vi "Sort Fcurve fxp.vi"(0 "reference in":refnum<class "Fcurve.lvclass">, 2 "Interleaved data in":fxp<+/-,27,5>[](array[numeric]), 5 "error in (no error)":errorcluster) -> (7 "Fcurve out":cluster{"X":dbl[], "Y":dbl[]}[](graph), 14 "reference out":refnum<class "Fcurve.lvclass">, 16 "Interleaved data out":fxp<+/-,27,5>[](array[numeric]), 19 "error out":errorcluster)   [LabVIEW 2019, in "Fcurve.lvclass"]
doc: "Sorts interleaved data into Fcurve"
uses:
  Fcurve.lvclass
  TDMS_DataHandler_class/property name combo box.ctl
  TDMS_DataHandler_class/TDMS_DataHandler.lvclass
panel:
  out "Ret_in":i32
  out "Con_in":i32
  out "App_in":i32
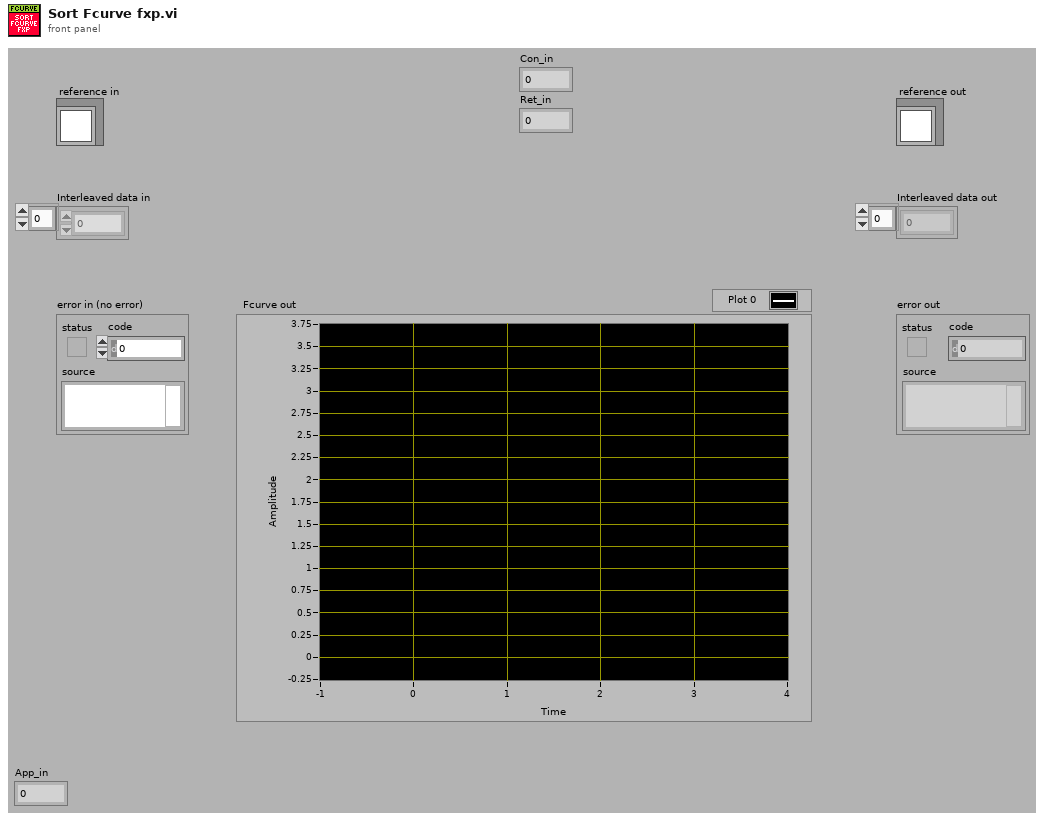
[diagram p1: front panel]
types:
  T1 = typedef "TDMS_DataHandler.lvclass/property name combo box.ctl" = string
  T2 = typedef "Fcurve.lvclass/ObjectAttributes.ctl" = cluster{"MyAttribute":dbl, "Fcurve Metadata":T3, "Contact Spread of dev":dbl, "Tau Delay (ms)":dbl, "Points of contact":dbl, "Def_wfm":cluster{"Max":dbl, "Min":dbl}, "Zpos_wfm":cluster{"Max":dbl, "Min":dbl}, "Contact stat?":bool, "Real AI dt (s)":dbl, "Decimation":cluster{"App":cluster{"Dec":i32, "apply":bool}, "Con":cluster{"Dec":i32, "apply":bool}, "Ret":cluster{"Dec":i32, "apply":bool}}, "Segment def[0]":dbl, "Segment Zpos[0]":dbl, "Raw Datum":waveform(dbl)[], "Group metadata":T4, "M_data obj":refnum<class "metadata.lvclass">, "Channel name(s)":string[], "Segment fcurve data":cluster{"X":dbl[], "Y":dbl[]}[], "Segment duration":cluster{"Start":i32, "Duration":i32}[], "Segment info":T5[], "Segment durations (S)":dbl[], "Segments Maxmin":T7[]}
  T3 = typedef "Fcurve.lvclass/Metadata.ctl" = cluster{"dt (us)":dbl, "Dec Factor":dbl, "Z piezo Sensitivity (nm/V)":dbl, "K (N/m)":dbl, "Sp (V)":dbl, "Contact (ms)":dbl, "Zpos contact":dbl, "Vel_app (nm/s)":dbl, "Vel_ret (nm/s)":dbl, "deltaV (nm)":dbl, "Def_V0 (v)":dbl, "Piezo gain":dbl, "invOLS (nm/V)":dbl}
  T4 = typedef "TDMS_DataHandler.lvclass/Fcurve Meta data.ctl" = cluster{"property names":string[], "property values":variant[]}
  T5 = typedef "Fcurve.lvclass/Fcurve segments --cluster.ctl" = cluster{"type":T6, "nb points":i32, "dec factor":u32, "sampling rate (S/s)":u32}
  T6 = typedef "metadata.lvclass/Segment type--combobox.ctl" = string
  T7 = typedef "Fcurve.lvclass/Segment MaxMin --cluster.ctl" = cluster{"Def":cluster{"max value":dbl, "min value":dbl}, "Zpos":cluster{"max value":dbl, "min value":dbl}}
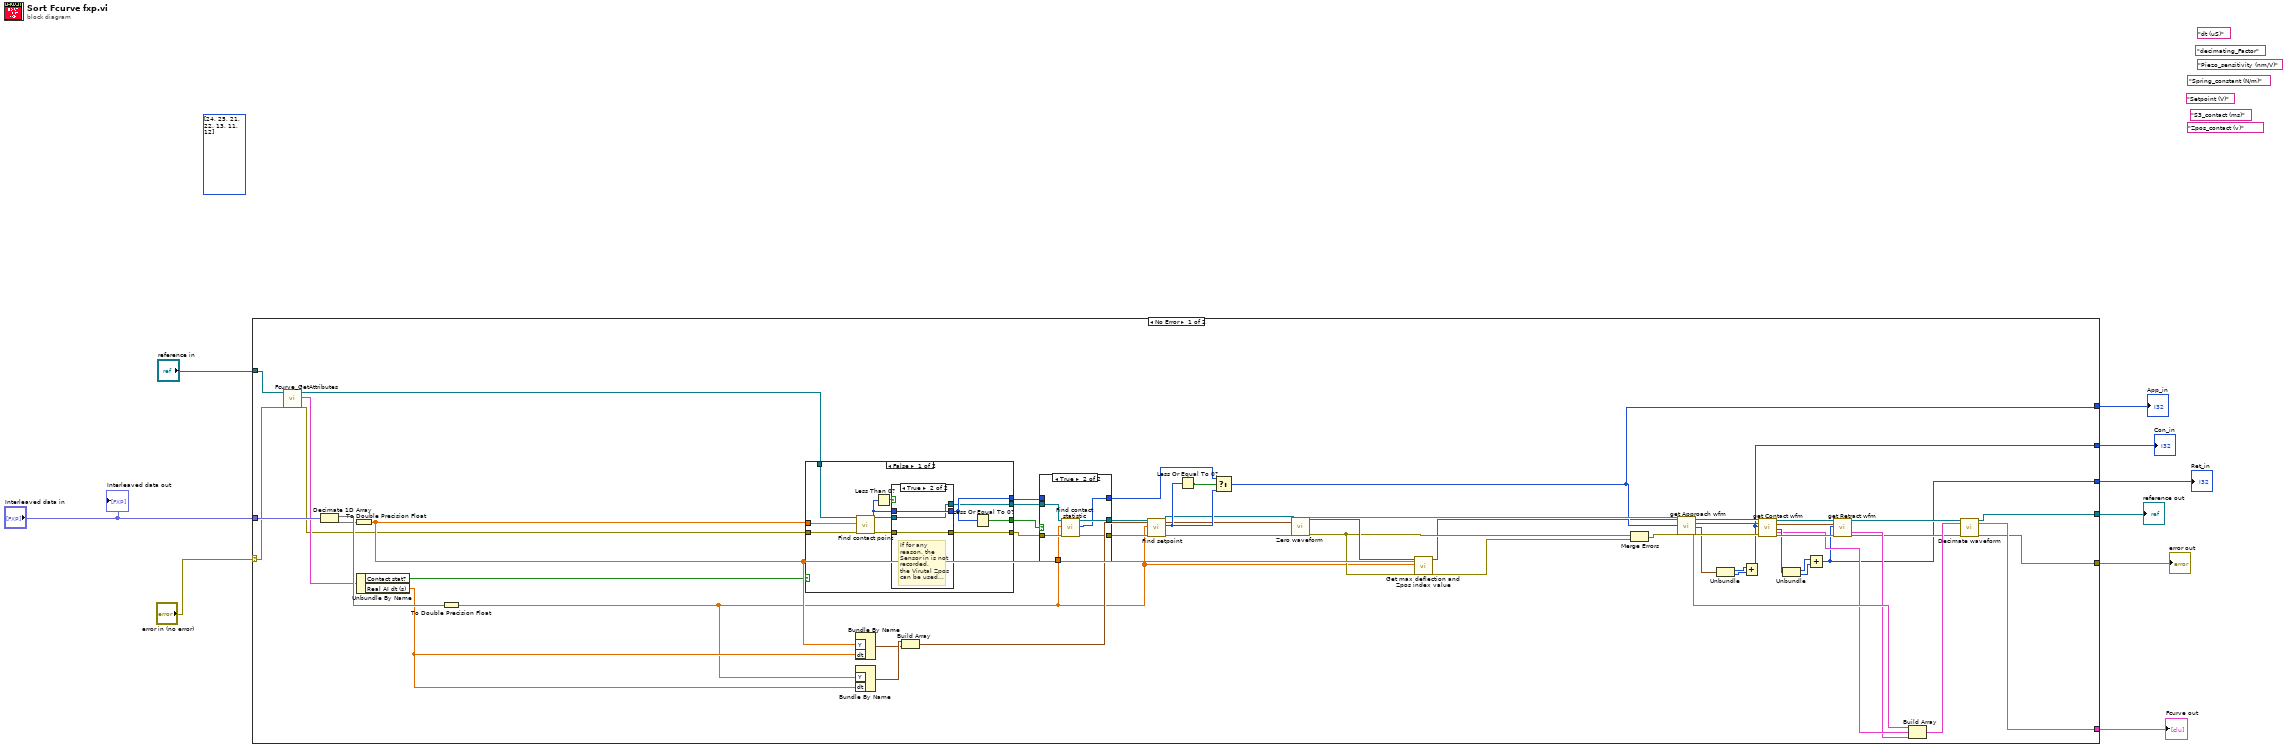
[diagram p0: block diagram]
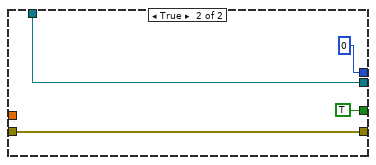
[diagram p3: hidden frame]
diagram:
  (unwired) i32[] [24, 25, 21, 22, 13, 11, 12] ("Array")
  (unwired) T1 "Setpoint (V)" ("Combo Box")
  (unwired) T1 "S3_contact (ms)" ("Combo Box")
  (unwired) T1 "Zpos_contact (v)" ("Combo Box")
  (unwired) T1 "Spring_constant (N/m)" ("Combo Box")
  (unwired) T1 "Piezo_sensitivity (nm/V)" ("Combo Box")
  (unwired) T1 "decimating_Factor" ("Combo Box")
  (unwired) T1 "dt (uS)" ("Combo Box")
  n1 = case shown="No Error" "error in (no error)" {
    selector: "error in (no error)" -> [w47 w96]
    tunnel: "Interleaved data in" -> [w64 _]
    tunnel: "reference in" -> [w61 w97]
    tunnel: [w23 w97] -> w7
    tunnel: [w19 w96] -> w6
    tunnel: [w21 _] -> w4
    tunnel: [w16 _] -> w3
    tunnel: [w15 _] -> w2
    tunnel: [w14 _] -> w1
    frame No Error {
      n2 = call "Fcurve_GetAttributes.vi"("reference in"=w61, "error in (no error)"=w47) -> ("reference out"=w28:refnum<class "Fcurve.lvclass">, "attributes"=w60:T2, "error out"=w18:errorcluster)  [unwired: 14 in, 1 out]
      n3 = Decimate 1D Array(w64) -> (w63:fxp<+/-,27,5>[], w62:fxp<+/-,27,5>[])
      n4 = To Double Precision Float(number=w62) -> (double precision float=w40:dbl[])
      n5 = Unbundle By Name(w60) -> ("Contact stat?"=w26:bool, "Real AI dt (s)"=w17:dbl)
      n6 = To Double Precision Float(number=w63) -> (double precision float=w10:dbl[])
      n7 = case shown="False" w26 {
        tunnel: [w68 TRUE] -> w33
        tunnel: [w69 0 ("Zpos index")] -> w65
        tunnel: w28 -> [w76 w83]
        tunnel: w40 -> [w75 _]
        tunnel: w18 -> [w74 w84]
        tunnel: [w72 w84] -> w59
        tunnel: [w66 w83] -> w58
        frame False {
          n8 = call "Find contact point.vi"("reference in"=w76, "Z pos (V)"=w75, "error in (no error)"=w74) -> ("reference out"=w67:refnum<class "Fcurve.lvclass">, "contact index"=w70:i32, "error out"=w71:errorcluster)  [unwired: 14 in]
          n9 = Less Than 0?(x=w70) -> (x < 0?=w73:bool)
          n10 = case shown="True" w73 {
            tunnel: [w79 w82] -> w72
            tunnel: w71 -> [w79 w82]
            tunnel: [w78 w81] -> w69
            tunnel: w70 -> [w78 w81]
            tunnel: w67 -> [w77 w80]
            tunnel: [w77 w80] -> w66
            frame False {
            }
            frame True {
              # "If for any reason, the Sensor in is not recorded,\nthe Virutal Zpos can be used..."
            }
          }
          n11 = Less Or Equal To 0?(x=w69) -> (x <= 0?=w68:bool)
        }
        frame True {
        }
      }
      n12 = Bundle By Name("Y"=w40, "dt"=w17) -> (w37:waveform(dbl))  [unwired: 1 in]
      n13 = Bundle By Name("Y"=w10, "dt"=w17) -> (w38:waveform(dbl))  [unwired: 1 in]
      n14 = Build Array(w38, w37) -> (w25:waveform(dbl)[])
      n15 = case shown="True" w33 {
        tunnel: [w87 w93] -> w57
        tunnel: [w89 w94] -> w45
        tunnel: w65 -> [w89 _]
        tunnel: [w88 w95] -> w56
        tunnel: w59 -> [w87 w92]
        tunnel: w58 -> [w88 w91]
        tunnel: w10 -> [_ w90]
        frame False {
        }
        frame True {
          n16 = call "Find contact statistic.vi"("reference in"=w91, "Deflection (V)"=w90, "error in (no error)"=w92) -> ("reference out"=w95:refnum<class "Fcurve.lvclass">, "contact point index out"=w94:i32, "error out"=w93:errorcluster)  [unwired: 14 in]
        }
      }
      n17 = call "Find setpoint.vi"("reference in"=w56, "Deflection"=w10, "error in (no error)"=w57) -> ("reference out"=w27:refnum<class "Fcurve.lvclass">, "Setpoint index"=w44:i32, "error out"=w42:errorcluster)  [unwired: 14 in]
      n18 = Less Or Equal To 0?(x=w44) -> (x <= 0?=w46:bool)
      n19 = Select(t=w45, s=w46, f=w44) -> (s? t:f=w14:i32)
      n20 = call-dynamic "Zero waveform.vi"("reference in"=w27, 1:w25, "error in (no error)"=w42) -> ("reference out"=w13:refnum<class "Fcurve.lvclass">, 15:w43, "error out"=w12:errorcluster)  [unwired: 11 in, 3 out]
      n21 = call "Get max deflection and Zpos index value.vi"("reference in"=w13, ">Zpos (V): Sensor IN>"=w40, ">Deflection (V)>"=w10, "error in (no error)"=w12) -> ("reference out"=w11:refnum<class "Fcurve.lvclass">, "error out"=w41:errorcluster)  [unwired: 14 in]
      n22 = Merge Errors(w12, w41) -> (w39:errorcluster)
      n23 = call-dynamic "get Approach wfm.vi"("reference in"=w11, "Zeroed (wfms.array)"=w43, 2:w14, "error in (no error)"=w39) -> ("reference out"=w53:refnum<class "Fcurve.lvclass">, "Zeroed (wfms.array) out"=w55:waveform(dbl)[], "Index [start,duration]"=w49:cluster{"Start":i32, "Duration":i32}, "Approach"=w36:cluster{"X":dbl[], "Y":dbl[]}, "error out"=w51:errorcluster)  [unwired: 10 in, 1 out]
      n24 = Unbundle(w49) -> ("Start"=w30:i32, "Duration"=w29:i32)
      n25 = Add(x=w30, y=w29) -> (x+y=w15:i32)
      n26 = call-dynamic "get Contact wfm.vi"("reference in"=w53, ".Zeroed (wfms.array)"=w55, "End Index (approach)"=w15, "error in (no error)"=w51) -> ("reference out"=w52:refnum<class "Fcurve.lvclass">, "Zeroed (wfms.array) out"=w54:waveform(dbl)[], "Contact indices [start,duration]"=w48:cluster{"Start":i32, "Duration":i32}, "Contact"=w35:cluster{"X":dbl[], "Y":dbl[]}, "error out"=w50:errorcluster)  [unwired: 10 in, 1 out]
      n27 = Unbundle(w48) -> ("Start"=w32:i32, "Duration"=w31:i32)
      n28 = Add(x=w32, y=w31) -> (x+y=w16:i32)
      n29 = call-dynamic "get Retract wfm.vi"("reference in"=w52, "Zeroed (wfms.array)"=w54, "End contact (index)"=w16, "error in (no error)"=w50) -> ("reference out"=w24:refnum<class "Fcurve.lvclass">, "Retract"=w34:cluster{"X":dbl[], "Y":dbl[]}, "error out"=w20:errorcluster)  [unwired: 10 in, 3 out]
      n30 = Build Array(w36, w35, w34) -> (w22:cluster{"X":dbl[], "Y":dbl[]}[])
      n31 = call-dynamic "Decimate waveform.vi"("reference in"=w24, 1:w22, "error in (no error)"=w20) -> ("reference out"=w23:refnum<class "Fcurve.lvclass">, "Decimated Fcurve (App,Con,Ret)"=w21:cluster{"X":dbl[], "Y":dbl[]}[], "error out"=w19:errorcluster)  [unwired: 14 in]
    }
    frame Error {
    }
  }
  "error out" <- w6
  "reference out" <- w7
  "Fcurve out" <- w4
  "App_in" <- w1
  "Con_in" <- w2
  "Ret_in" <- w3
  "Interleaved data out" <- "Interleaved data in"
